vi "Contour Page.vi"() -> ()   [LabVIEW 2020, in "3D Contour.lvclass"]
uses:
  <vilib>/Math Plots/3D Math Plots/3D Contour/3D Contour/3D Contour.lvclass
  <vilib>/Math Plots/3D Math Plots/3D Contour/3D Contour/Typedef/3D Contour Property Array.ctl
  <vilib>/Math Plots/3D Math Plots/3D Contour/3D Contour/Typedef/3D Contour Property.ctl
  <vilib>/Math Plots/3D Math Plots/3D Plot/3D Plot/Typedef/Line Type.ctl
  <vilib>/Math Plots/3D Math Plots/3D Plot/3D Plot/Typedef/Color Ramp Cluster.ctl
  <vilib>/Math Plots/3D Math Plots/3D Plot/3D Plot/Typedef/Dialog State.ctl
  <vilib>/Math Plots/3D Math Plots/3D Plot/3D Plot/Typedef/Temp Scene State.ctl
  <vilib>/Math Plots/3D Math Plots/3D Plot/3D Plot/Typedef/Temp Scene Property Action.ctl
  <vilib>/Math Plots/3D Math Plots/3D Plot/3D Plot/3D Plot.lvclass
panel:
  out "Contour Property Out":T1
  in  "Contour Property In":T1
  in  "Interval":sgl min=0 step=0.001
  in  "Line Style":u16(ring) caption="Line style"
  in  "Antialiasing":bool
  in  "Line Width":sgl=0.001 caption="Line width" min=0.001 step=1
  in  "Line Color":u32(colorbox) caption="Line color"
  in  "Contour Mode":u16(ring) caption="Contour mode" items=["Contour", "Contour with surface"]
  in  "Axis Basis":u16(ring) caption="Axis basis" items=["X-Axis", "Y-Axis", "Z-Axis"]
  in  "Levels":u16=1 min=1 step=1
  in  "Level List":i32(listbox) caption="Level list"
  in  "Level Mode":u16(ring) caption="Level mode" items=["Levels", "Interval", "Level List"]
  in  "Ramp Edit":bool caption="Ramp edit"
  in  "Color Map Style":u16(ring) caption="Color map style" items=["None ", "Shaded", "Color spectrum", "Grey scale", "Custom"]
  out "Color Ramp":dbl[][](graph)
  in  "YZ Plane Projection":bool caption="YZ plane projection"
  in  "XZ Plane Projection":bool caption="XZ plane projection"
  in  "XY Plane Projection":bool caption="XY  plane projection"
  in  "Coordinate System":u16(ring) caption="Coordinate system" items=["Cartesian", "Cylindrical", "Spherical"]
  in  "Plot Opacity":sgl(slide) caption="Plot opacity(%)" min=0 max=100 scale=0.0..100.0
  in  "New":bool
  in  "Delete":bool
  in  "Move Up":bool
  in  "Move Down":bool
  in  "Plot List":i32(listbox)
  in  "Level Conflict":string="Can't have two contours have the same level."
  in  "New Line":string="[Add new level here]"
  in  "Event Registration":refnum<event-registration>
  # "Contour"
  # "General"
  # "Projection"
  # "Color Ramp"
  # "Contour"
  # "Line"
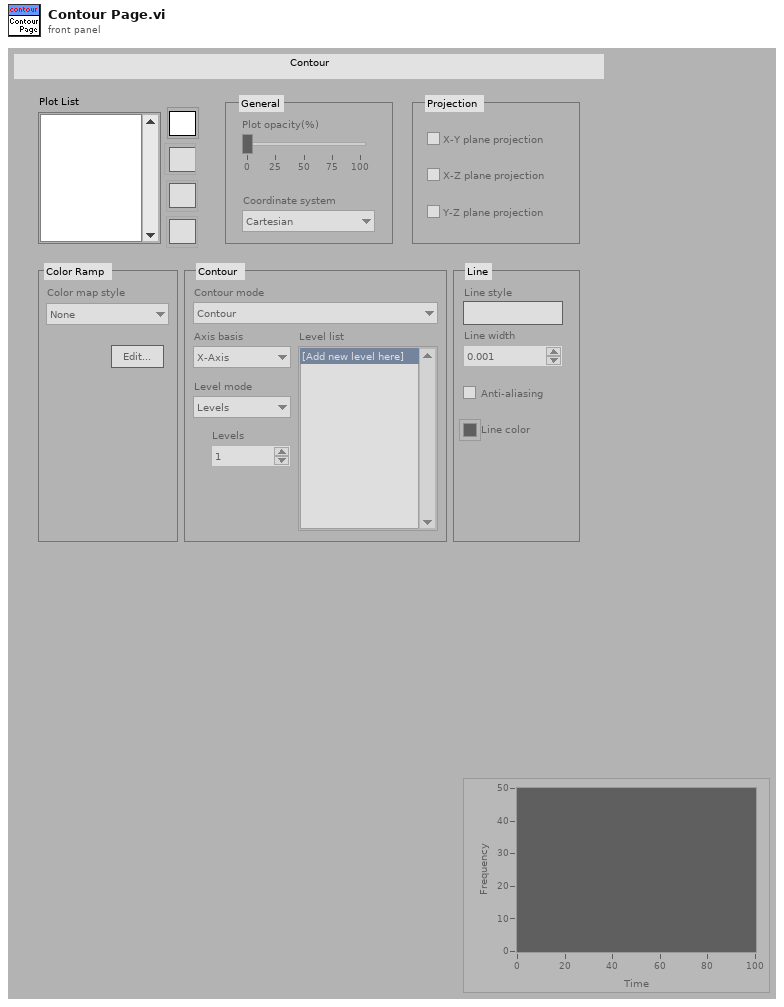
[diagram p1: front panel]
types:
  T1 = typedef "3D Contour.lvclass/3D Contour Property Array.ctl" = T2[]
  T2 = typedef "3D Contour.lvclass/3D Contour Property.ctl" = cluster{"General Property":cluster{"Plot Name":string, "Coordinate System":enum16{"Cartesian", "Cylindrical", "Spherical"}, "Opacity":sgl}, "Projection Property":cluster{"Draw XY":bool, "Draw YZ":bool, "Draw XZ":bool}, "Plot Property":cluster{"Line Style":T3, "Line Width":sgl, "Line Color":u32, "Antialiasing":bool, "Color Ramp Cluster":T4}, "Contour Property":cluster{"Contour Type":enum16{"Contour", "Contour with surface"}, "Axis Basis":enum16{"X-Axis", "Y-Axis", "Z-Axis"}, "Level List":sgl[], "Level Mode":enum16{"Levels", "Interval", "Level List"}, "Levels":u16, "Interval":sgl}}
  T3 = typedef "3D Plot.lvclass/Line Type.ctl" = enum16{"None", "Solid", "Dash", "Dot", "Dash Dot"}
  T4 = typedef "3D Plot.lvclass/Color Ramp Cluster.ctl" = cluster{"Color Ramp Style":enum16{"None", "Shaded", "Color spectrum", "Grey scale", "Custom"}, "Color Ramp Array":u32[], "Color Ramp Index":i32[], "Interpolate?":bool, "Logarithm?":bool}
  T5 = typedef "3D Plot.lvclass/Dialog State.ctl" = enum16{"Initialize", "Read Porperty", "Write Property", "Idle", "Exit"}
  T6 = typedef "3D Plot.lvclass/Temp Scene State.ctl" = enum16{"Create", "Update Scene", "Get Plot Representation", "Destory"}
  T7 = typedef "3D Plot.lvclass/Temp Scene Property Action.ctl" = enum16{"Graph Property", "Light Property", "Axis Property", "Value Pair Property", "Format Property", "Cursor Property", "Plot Specific Property"}
  T8 = typedef "3D Plot.lvclass/Multiplot Representation.ctl" = cluster{"Plot Represention Array":T9[], "Max Range":T10}
  T9 = typedef "3D Plot.lvclass/Plot Representation.ctl" = cluster{"Plot ID":i32, "Plot Range":T10, "Mesh Data":T11, "Dimension":cluster{"X Dimension":i32, "Y Dimension":i32}, "Ramp Range":T10}
  T10 = typedef "3D Plot.lvclass/Range Clusters.ctl" = cluster{"X Range":cluster{"Max X":sgl, "Min X":sgl}, "Y Range":cluster{"Max Y":sgl, "Min Y":sgl}, "Z Range":cluster{"Max Z":sgl, "Min Z":sgl}}
  T11 = typedef "3D Plot.lvclass/Mesh Data.ctl" = cluster{"Index Array":u32[], "Vertex Array":cluster{"X":sgl, "Y":sgl, "Z":sgl}[], "Normal Array":cluster{"X":sgl, "Y":sgl, "Z":sgl}[], "Color Index Array":i32[]}
  T12 = enum16{"None", "Shaded", "Color spectrum", "Grey scale", "Custom"}
  T13 = typedef "eventvkey.ctl" = enum16{"ASCII", "Enter", "Return", "Shift", "Ctrl", "Alt", "Cmd", "Opt", "Caps", "NumLock", "Clear", "Break", "Up", "Down", "Left", "Right", "Insert", "Delete", "Home", "End", "PageUp", "PageDown", "Escape", "Help", "Pause", "ScrollLock", "F1", "F2", "F3", "F4", "F5", "F6", "F7", "F8", "F9", "F10", "F11", "F12", "F13", "F14", "F15", "F16", "F17", "F18", "F19", "F20", "F21", "F22", "F23", "F24", "Play", "VolumeUp", "VolumeDown", "Mute", "Two Byte Char"}
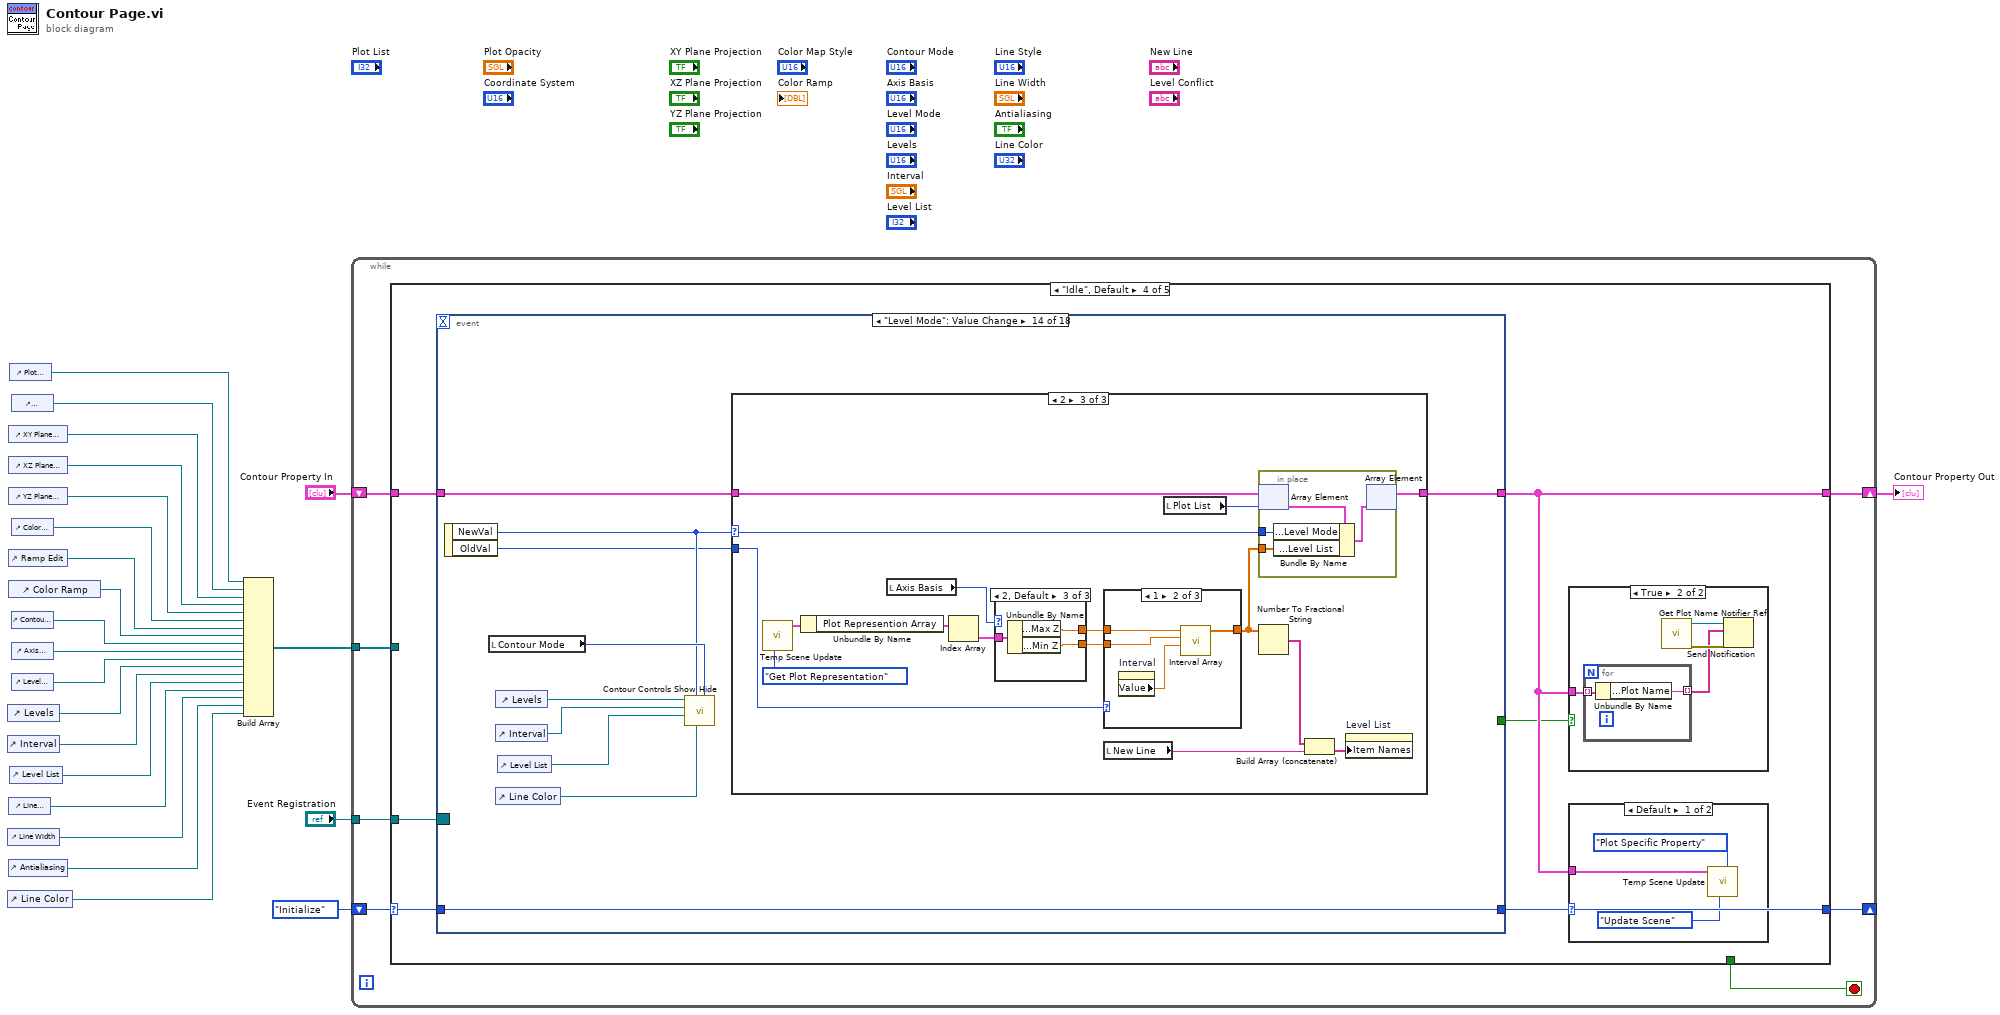
[diagram p0: block diagram]
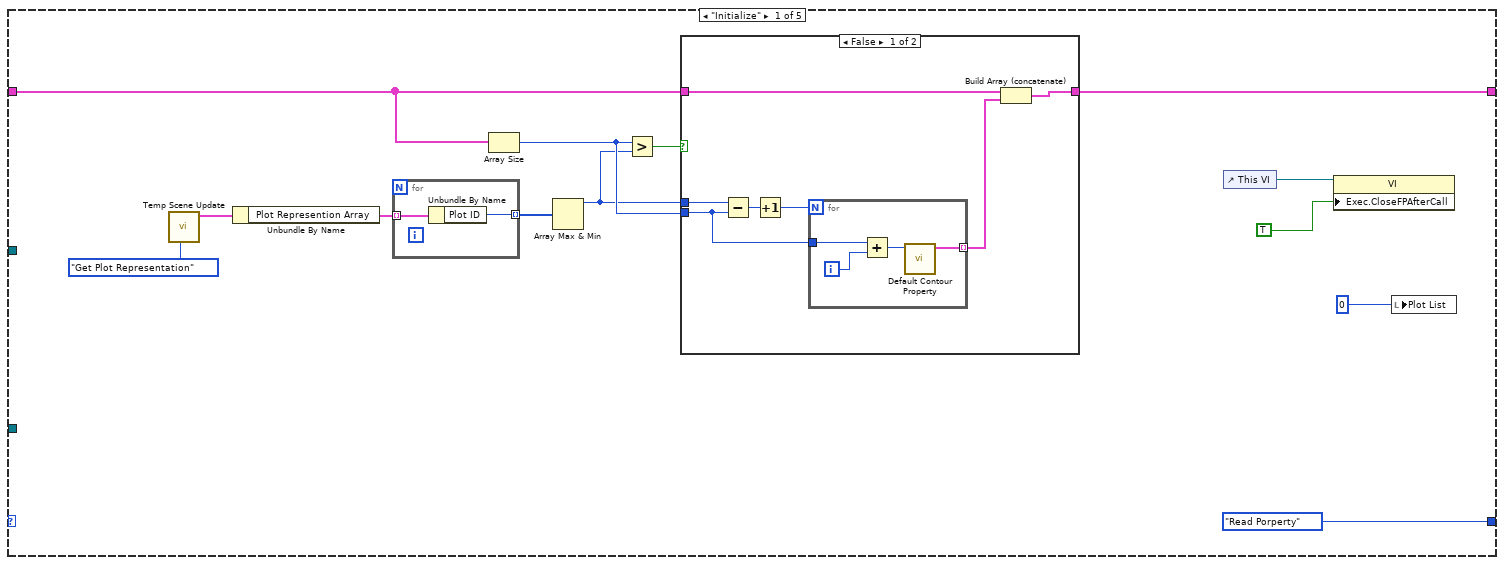
[diagram p2: hidden frame]
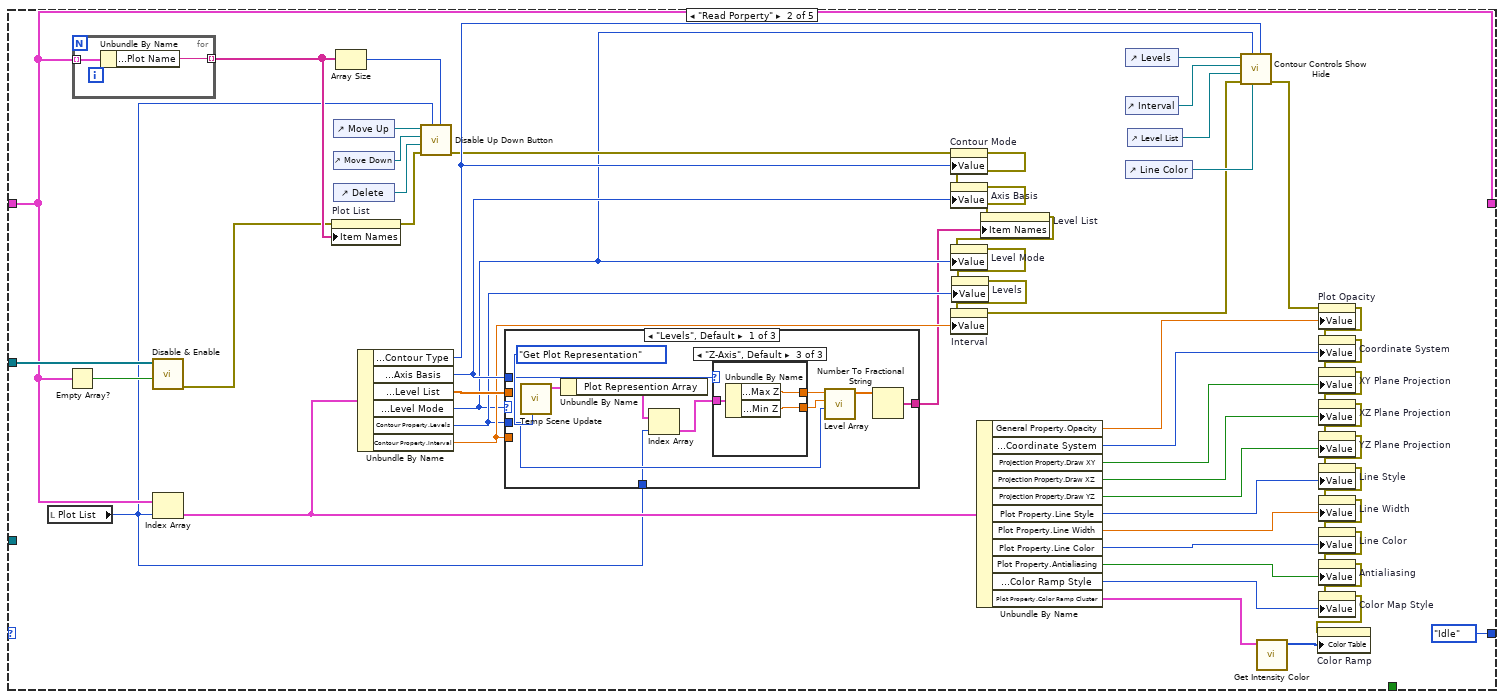
[diagram p4: hidden frame]
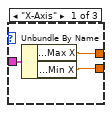
[diagram p5: hidden frame]
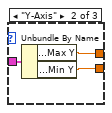
[diagram p6: hidden frame]
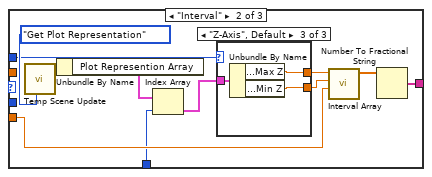
[diagram p7: hidden frame]
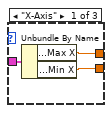
[diagram p8: hidden frame]
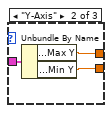
[diagram p9: hidden frame]
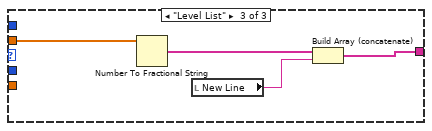
[diagram p10: hidden frame]
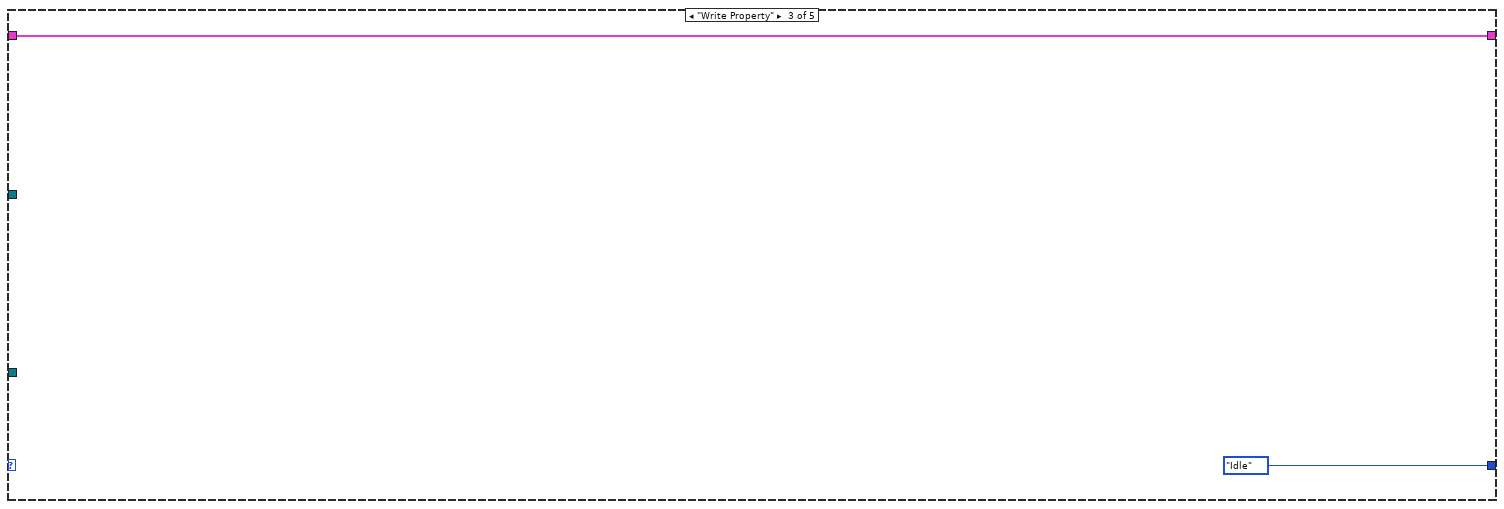
[diagram p11: hidden frame]
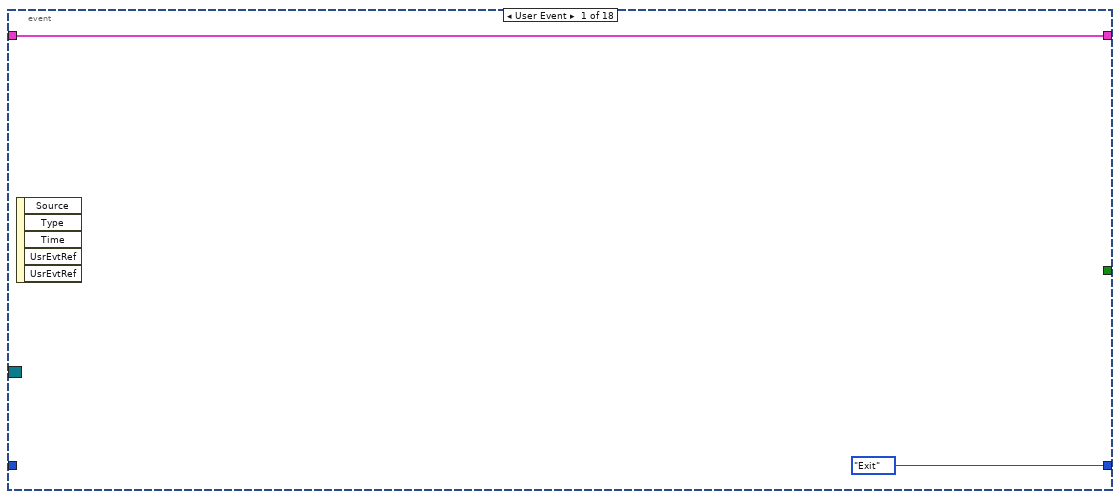
[diagram p14: hidden frame]
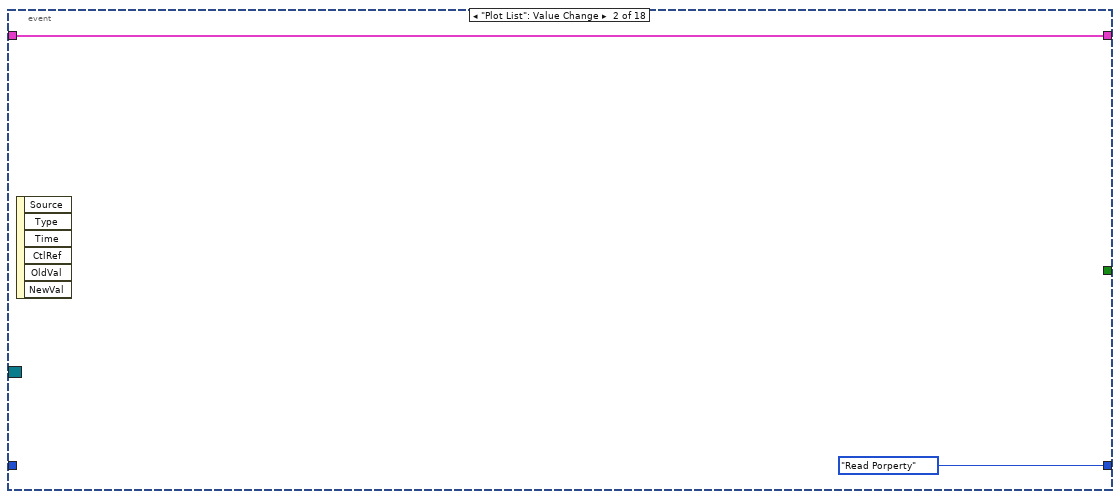
[diagram p15: hidden frame]
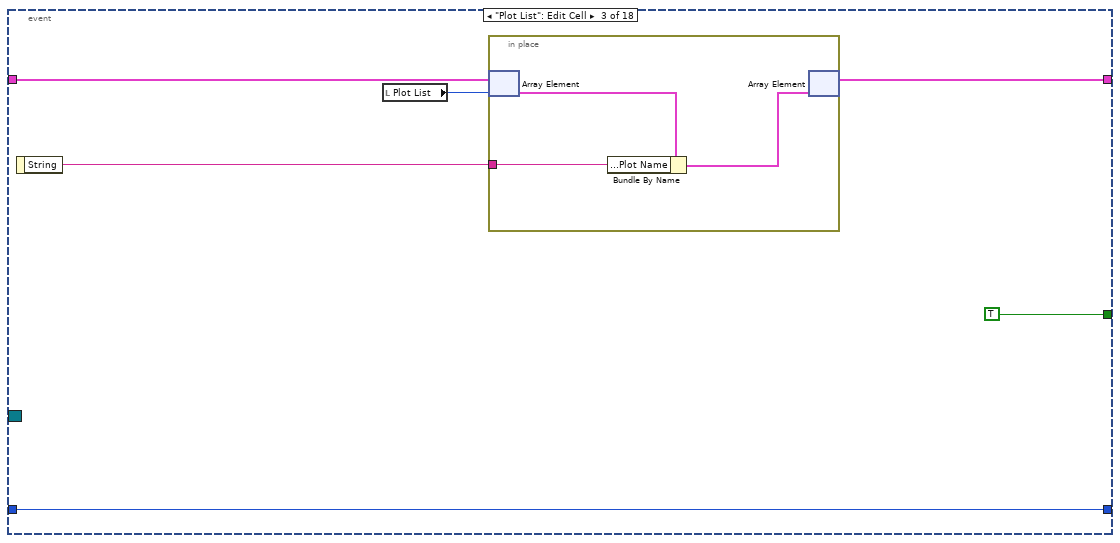
[diagram p16: hidden frame]
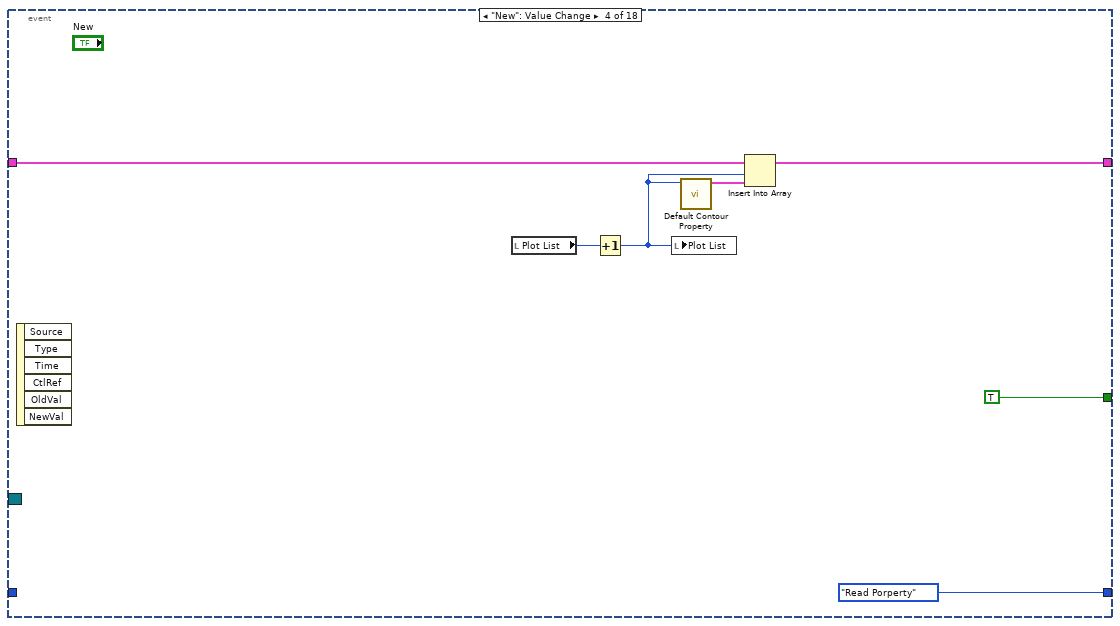
[diagram p17: hidden frame]
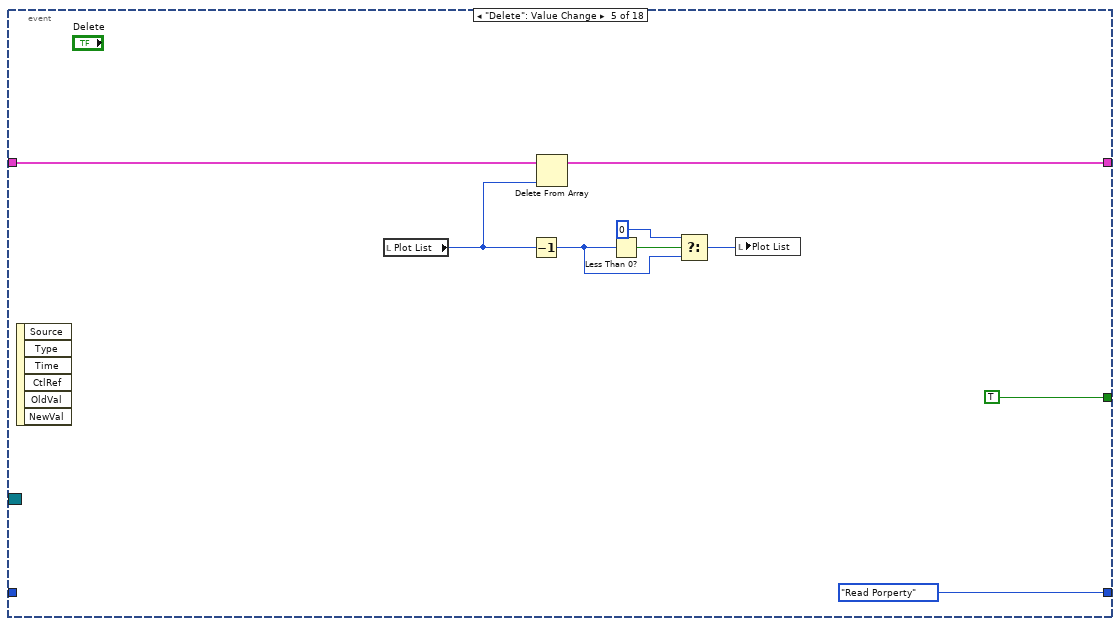
[diagram p18: hidden frame]
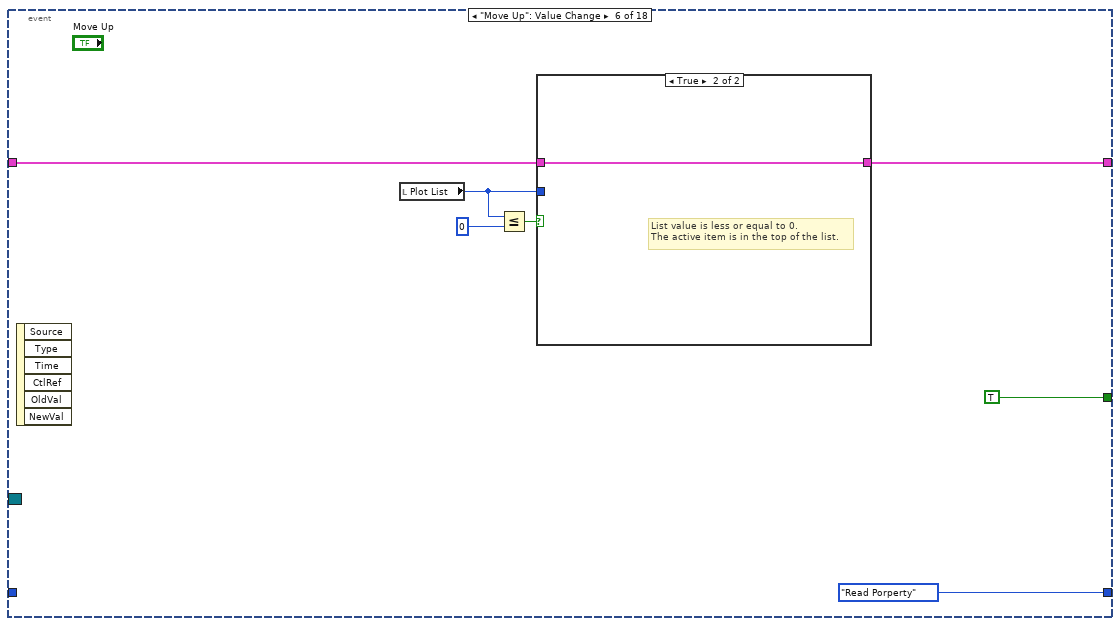
[diagram p19: hidden frame]
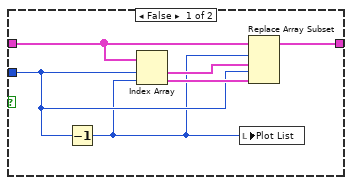
[diagram p20: hidden frame]
diagram:
  n1 = control-ref of="Levels"() -> (w8:refnum<vi>)
  n2 = control-ref of="Interval"() -> (w7:refnum<vi>)
  n3 = control-ref of="Line Width"() -> (w4:refnum<vi>)
  n4 = control-ref of="Line Color"() -> (w2:refnum<vi>)
  n5 = control-ref of="XY Plane Projection"() -> (w17:refnum<vi>)
  n6 = control-ref of="XZ Plane Projection"() -> (w16:refnum<vi>)
  n7 = control-ref of="YZ Plane Projection"() -> (w15:refnum<vi>)
  n8 = control-ref of="Ramp Edit"() -> (w13:refnum<vi>)
  n9 = control-ref of="Color Ramp"() -> (w12:refnum<vi>)
  n10 = control-ref of="Line Style"() -> (w5:refnum<vi>)
  n11 = control-ref of="Antialiasing"() -> (w3:refnum<vi>)
  n12 = control-ref of="Plot Opacity"() -> (w19:refnum<vi>)
  n13 = control-ref of="Level List"() -> (w6:refnum<vi>)
  n14 = control-ref of="Coordinate System"() -> (w18:refnum<vi>)
  n15 = control-ref of="Color Map Style"() -> (w14:refnum<vi>)
  n16 = control-ref of="Contour Mode"() -> (w11:refnum<vi>)
  n17 = control-ref of="Axis Basis"() -> (w10:refnum<vi>)
  n18 = control-ref of="Level Mode"() -> (w9:refnum<vi>)
  n19 = Build Array(w19, w18, w17, w16, w15, w14, w13, w12, w11, w10, w9, w8, w7, w6, w5, w4, w3, w2) -> (w1:refnum<vi>[])
  n20 = while {
    shift-right: [w29] -> w20
    shift-left: "Contour Property In" -> [w30]
    shift-right: [w25] -> _
    shift-left: Dialog_State."Initialize" -> [w28]
    tunnel: "Event Registration" -> [w26]
    tunnel: w1 -> [w24]
    stop <- w27 stop-if-true
    n21 = case shown="\"Idle\", Default" w28 {
      selector: w28 -> [_ _ _ w163 _]
      tunnel: w30 -> [w33 w96 w158 w165 w606]
      tunnel: [w32 w96 w158 w161 w606] -> w29
      tunnel: [Dialog_State."Read Porperty" Dialog_State."Idle" Dialog_State."Idle" w162 Dialog_State."Exit"] -> w25
      tunnel: [_ _ _ _ TRUE] -> w27
      tunnel: w26 -> [_ _ _ w164 _]
      tunnel: w24 -> [_ w97 _ _ _]
      frame "Initialize" {
        n22 = call <vilib>:"Temp Scene Update.vi"("State"=Temp_Scene_State."Get Plot Representation") -> ("Multiplot Representation"=w38:T8)  [unwired: 5 in, 5 out]
        n23 = Unbundle By Name(w38) -> ("Plot Represention Array"=w31:T9[])
        n24 = for {
          tunnel: w31 -> [w57] mode=indexing
          tunnel: [w56] -> w37 mode=indexing
          n25 = Unbundle By Name(w57) -> ("Plot ID"=w56:i32)
        }
        n26 = Array Size(array=w33) -> (size(s)=w35:i32)
        n27 = Array Max & Min(array=w37) -> (max value=w34:i32)  [unwired: 3 out]
        n28 = Greater?(x=w35, y=w34) -> (0:w36:bool)
        n29 = case shown="False" w36 {
          tunnel: [w48 w55] -> w32
          tunnel: w33 -> [w50 w55]
          tunnel: w35 -> [w44 _]
          tunnel: w34 -> [w45 _]
          frame False {
            n30 = Subtract(x=w45, y=w44) -> (x-y=w47:i32)
            n31 = Increment(x=w47) -> (x+1=w46:i32)
            n32 = for {
              N: w46 -> [_]
              tunnel: w44 -> [w53]
              tunnel: [w51] -> w49 mode=indexing
              i -> [w54]
              n33 = Add(x=w53, y=w54) -> (x+y=w52:i32)
              n34 = call <vilib>:"Default Contour Property.vi"("Plot ID"=w52) -> ("Default Property"=w51:T2)  [unwired: 10 out]
            }
            n35 = Build Array (concatenate)(w50, w49) -> (w48:T1)
          }
          frame True {
          }
        }
        n36 = control-ref of="This VI"() -> (w42:refnum<vi>)
        n37 = property class="VI"(reference=w42, "Exec.CloseFPAfterCall"=TRUE ("Execution:Close After Call")) -> ()  [unwired: 1 in, 2 out]
        n38 = local write "Plot List"(0 ("Plot List")) -> ()
      }
      frame "Read Porperty" {
        n39 = local read "Plot List"() -> (w59:i32)
        n40 = Empty Array?(array=w96) -> (empty?=w98:bool)
        n41 = for {
          tunnel: w96 -> [w157] mode=indexing
          tunnel: [w156] -> w104 mode=indexing
          n42 = Unbundle By Name(w157) -> ("General Property.Plot Name"=w156:string)
        }
        n43 = call <vilib>:"Disable & Enable.vi"("Disabled?"=w98, "Control Ref Array"=w97) -> ("error out"=w95:errorcluster)  [unwired: 1 in, 8 out]
        n44 = Index Array(array=w96, index=w59) -> (element=w110:T2)
        n45 = property on="Plot List" class="LstBox (strict)"(error in=w95, "Item Names"=w104) -> (error out=w103:errorcluster)  [unwired: 1 in, 1 out]
        n46 = control-ref of="Move Up"() -> (w106:refnum<vi>)
        n47 = control-ref of="Move Down"() -> (w107:refnum<vi>)
        n48 = control-ref of="Delete"() -> (w108:refnum<vi>)
        n49 = Array Size(array=w104) -> (size(s)=w105:i32)
        n50 = Unbundle By Name(w110) -> ("Contour Property.Contour Type"=w83:enum16{"Contour", "Contour with surface"}, "Contour Property.Axis Basis"=w64:enum16{"X-Axis", "Y-Axis", "Z-Axis"}, "Contour Property.Level List"=w65:sgl[], "Contour Property.Level Mode"=w61:enum16{"Levels", "Interval", "Level List"}, "Contour Property.Levels"=w62:u16, "Contour Property.Interval"=w63:sgl)
        n51 = call <vilib>:"Disable Up Down Button.vi"("Length"=w105, "Index"=w59, "error in (no error)"=w103, "Delete Ref"=w108, "Move Down Ref"=w107, "Move Up Ref"=w106) -> ("error out"=w69:errorcluster)  [unwired: 5 out]
        n52 = case shown="\"Levels\", Default" w61 {
          tunnel: [w114 w134 w152] -> w60
          tunnel: w65 -> [_ _ w155]
          tunnel: w64 -> [w117 w137 _]
          tunnel: w63 -> [_ w136 _]
          tunnel: w62 -> [w116 _ _]
          tunnel: w59 -> [w113 w133 _]
          frame "Levels", Default {
            n53 = call <vilib>:"Temp Scene Update.vi"("State"=Temp_Scene_State."Get Plot Representation") -> ("Multiplot Representation"=w118:T8)  [unwired: 5 in, 5 out]
            n54 = Unbundle By Name(w118) -> ("Plot Represention Array"=w112:T9[])
            n55 = Index Array(array=w112, index=w113) -> (element=w120:T9)
            n56 = case shown="\"Z-Axis\", Default" w117 {
              tunnel: w120 -> [w125 w128 w131]
              tunnel: [w124 w127 w130] -> w122
              tunnel: [w123 w126 w129] -> w121
              frame "X-Axis" {
                n57 = Unbundle By Name(w125) -> ("Plot Range.X Range.Max X"=w124:sgl, "Plot Range.X Range.Min X"=w123:sgl)
              }
              frame "Y-Axis" {
                n58 = Unbundle By Name(w128) -> ("Plot Range.Y Range.Max Y"=w127:sgl, "Plot Range.Y Range.Min Y"=w126:sgl)
              }
              frame "Z-Axis", Default {
                n59 = Unbundle By Name(w131) -> ("Plot Range.Z Range.Max Z"=w130:sgl, "Plot Range.Z Range.Min Z"=w129:sgl)
              }
            }
            n60 = call <vilib>:"Level Array.vi"("Level"=w116, "Min"=w121, "Max"=w122) -> ("Level Array"=w115:sgl[])  [unwired: 8 out]
            n61 = Number To Fractional String(number=w115) -> (F-format string=w114:string[])  [unwired: 3 out]
          }
          frame "Interval" {
            n62 = call <vilib>:"Temp Scene Update.vi"("State"=Temp_Scene_State."Get Plot Representation") -> ("Multiplot Representation"=w138:T8)  [unwired: 5 in, 5 out]
            n63 = Unbundle By Name(w138) -> ("Plot Represention Array"=w132:T9[])
            n64 = Index Array(array=w132, index=w133) -> (element=w140:T9)
            n65 = case shown="\"Z-Axis\", Default" w137 {
              tunnel: w140 -> [w145 w148 w151]
              tunnel: [w144 w147 w150] -> w142
              tunnel: [w143 w146 w149] -> w141
              frame "X-Axis" {
                n66 = Unbundle By Name(w145) -> ("Plot Range.X Range.Max X"=w144:sgl, "Plot Range.X Range.Min X"=w143:sgl)
              }
              frame "Y-Axis" {
                n67 = Unbundle By Name(w148) -> ("Plot Range.Y Range.Max Y"=w147:sgl, "Plot Range.Y Range.Min Y"=w146:sgl)
              }
              frame "Z-Axis", Default {
                n68 = Unbundle By Name(w151) -> ("Plot Range.Z Range.Max Z"=w150:sgl, "Plot Range.Z Range.Min Z"=w149:sgl)
              }
            }
            n69 = call <vilib>:"Interval Array.vi"("Interval"=w136, "Min"=w141, "Max"=w142) -> ("Level Array"=w135:sgl[])  [unwired: 8 out]
            n70 = Number To Fractional String(number=w135) -> (F-format string=w134:string[])  [unwired: 3 out]
          }
          frame "Level List" {
            n71 = Number To Fractional String(number=w155) -> (F-format string=w154:string[])  [unwired: 3 out]
            n72 = local read "New Line"() -> (w153:string)
            n73 = Build Array (concatenate)(w154, w153) -> (w152:string[])
          }
        }
        n74 = property on="Contour Mode" class="Ring (strict)"(error in=w69, "Value"=w83) -> (error out=w94:errorcluster)  [unwired: 1 in, 1 out]
        n75 = property on="Axis Basis" class="Ring (strict)"(error in=w94, "Value"=w64) -> (error out=w82:errorcluster)  [unwired: 1 in, 1 out]
        n76 = Unbundle By Name(w110) -> ("General Property.Opacity"=w81:sgl, "General Property.Coordinate System"=w80:enum16{"Cartesian", "Cylindrical", "Spherical"}, "Projection Property.Draw XY"=w79:bool, "Projection Property.Draw XZ"=w78:bool, "Projection Property.Draw YZ"=w77:bool, "Plot Property.Line Style"=w76:T3, "Plot Property.Line Width"=w75:sgl, "Plot Property.Line Color"=w74:u32, "Plot Property.Antialiasing"=w73:bool, "Plot Property.Color Ramp Cluster.Color Ramp Style"=w72:T12, "Plot Property.Color Ramp Cluster"=w58:T4)
        n77 = property on="Level List" class="LstBox (strict)"(error in=w82, "Item Names"=w60) -> (error out=w71:errorcluster)  [unwired: 1 in, 1 out]
        n78 = property on="Level Mode" class="Ring (strict)"(error in=w71, "Value"=w61) -> (error out=w93:errorcluster)  [unwired: 1 in, 1 out]
        n79 = property on="Levels" class="DigNum (strict)"(error in=w93, "Value"=w62) -> (error out=w92:errorcluster)  [unwired: 1 in, 1 out]
        n80 = property on="Interval" class="DigNum (strict)"(error in=w92, "Value"=w63) -> (error out=w70:errorcluster)  [unwired: 1 in, 1 out]
        n81 = control-ref of="Levels"() -> (w102:refnum<vi>)
        n82 = control-ref of="Interval"() -> (w101:refnum<vi>)
        n83 = control-ref of="Line Color"() -> (w99:refnum<vi>)
        n84 = control-ref of="Level List"() -> (w100:refnum<vi>)
        n85 = call <vilib>:"Contour Controls Show Hide.vi"("Contour Mode"=w83, "Line Color Ref"=w99, "Level Mode"=w61, "error in (no error)"=w70, "Level List Ref"=w100, "Interval Ref"=w101, "Levels Ref"=w102) -> ("error out"=w67:errorcluster)  [unwired: 4 out]
        n86 = call <vilib>:"Get Intensity Color.vi"("Color Ramp Cluster"=w58) -> ("Intensity Color"=w109:u32[])  [unwired: 4 in, 6 out]
        n87 = property on="Plot Opacity" class="Slide (strict)"(error in=w67, "Value"=w81) -> (error out=w91:errorcluster)  [unwired: 1 in, 1 out]
        n88 = property on="Coordinate System" class="Ring (strict)"(error in=w91, "Value"=w80) -> (error out=w90:errorcluster)  [unwired: 1 in, 1 out]
        n89 = property on="XY Plane Projection" class="Bool (strict)"(error in=w90, "Value"=w79) -> (error out=w89:errorcluster)  [unwired: 1 in, 1 out]
        n90 = property on="XZ Plane Projection" class="Bool (strict)"(error in=w89, "Value"=w78) -> (error out=w88:errorcluster)  [unwired: 1 in, 1 out]
        n91 = property on="YZ Plane Projection" class="Bool (strict)"(error in=w88, "Value"=w77) -> (error out=w87:errorcluster)  [unwired: 1 in, 1 out]
        n92 = property on="Line Style" class="Ring (strict)"(error in=w87, "Value"=w76) -> (error out=w86:errorcluster)  [unwired: 1 in, 1 out]
        n93 = property on="Line Width" class="DigNum (strict)"(error in=w86, "Value"=w75) -> (error out=w85:errorcluster)  [unwired: 1 in, 1 out]
        n94 = property on="Line Color" class="ColBox"(error in=w85, "Value"=w74) -> (error out=w84:errorcluster)  [unwired: 1 in, 1 out]
        n95 = property on="Antialiasing" class="Bool (strict)"(error in=w84, "Value"=w73) -> (error out=w68:errorcluster)  [unwired: 1 in, 1 out]
        n96 = property on="Color Map Style" class="Ring (strict)"(error in=w68, "Value"=w72) -> (error out=w66:errorcluster)  [unwired: 1 in, 1 out]
        n97 = property on="Color Ramp" class="IntGraph (strict)"(error in=w66, "Color Table"=w109) -> ()  [unwired: 1 in, 2 out]
      }
      frame "Write Property" {
      }
      frame "Idle", Default {
        n98 = event shown="[13] \"Level Mode\": Value Change" {
          selector: w164 -> [_ _ _ _ _ _ _ _ _ _ _ _ _ _ _ _ _ _]
          dyn-events: _ -> [_ _ _ _ _ _ _ _ _ _ _ _ _ _ _ _ _ _]
          timeout: _ -> [_ _ _ _ _ _ _ _ _ _ _ _ _ _ _ _ _ _]
          tunnel: w165 -> [w176 w178 w182 w192 w201 w206 w220 w234 w247 w266 w287 w303 w318 w353 w452 w477 w504 w563]
          tunnel: [w176 w178 w181 w191 w202 w205 w219 w233 w244 w265 w286 w302 w317 w352 w451 w478 w503 w562] -> w161
          tunnel: [Dialog_State."Exit" Dialog_State."Read Porperty" w180 Dialog_State."Read Porperty" Dialog_State."Read Porperty" Dialog_State."Read Porperty" Dialog_State."Read Porperty" w236 w248 w268 w289 w304 w319 w354 w457 w483 w505 w564] -> w162
          tunnel: w163 -> [_ _ w180 _ _ _ _ w236 w248 w268 w289 w304 w319 w354 w457 w483 w505 w564]
          tunnel: [_ _ TRUE TRUE TRUE TRUE TRUE _ _ _ _ _ _ _ _ _ _ _] -> w160
          event User Event {
            n99 = event-data() -> ()  [unwired: 6 out]
          }
          event "Plot List": Value Change {
            n100 = event-data() -> ()  [unwired: 7 out]
          }
          event "Plot List": Edit Cell {
            n101 = event-data() -> ("String"=w183:string)  [unwired: 1 out]
            n102 = local read "Plot List"() -> (w184:i32)
            n103 = in-place {
              in-place-border: w183 -> [w185]
              n104 = in-place-array #1(w182, w184) -> (w187:T2)
              n105 = Bundle By Name(cluster=w187, "General Property.Plot Name"=w185) -> (w186:T2)
              n106 = in-place-array #1(w186) -> (w181:T1)  [unwired: 1 out]
            }
          }
          event "New": Value Change {
            n107 = event-data() -> ()  [unwired: 7 out]
            n108 = local read "Plot List"() -> (w193:i32)
            n109 = Increment(x=w193) -> (x+1=w189:i32)
            n110 = local write "Plot List"(w189) -> ()
            n111 = call <vilib>:"Default Contour Property.vi"("Plot ID"=w189) -> ("Default Property"=w188:T2)  [unwired: 10 out]
            n112 = Insert Into Array(array=w192, index=w189, new element=w188) -> (w191:T1)
          }
          event "Delete": Value Change {
            n113 = event-data() -> ()  [unwired: 7 out]
            n114 = local read "Plot List"() -> (w197:i32)
            n115 = Decrement(x=w197) -> (x-1=w198:i32)
            n116 = Delete From Array(array=w201, index=w197) -> (array with subset deleted=w202:T1)  [unwired: 1 in, 1 out]
            n117 = Less Than 0?(x=w198) -> (x < 0?=w200:bool)
            n118 = Select(t=0, s=w200, f=w198) -> (s? t:f=w196:i32)
            n119 = local write "Plot List"(w196) -> ()
          }
          event "Move Up": Value Change {
            n120 = event-data() -> ()  [unwired: 7 out]
            n121 = local read "Plot List"() -> (w207:i32)
            n122 = Less Or Equal?(x=w207, y=0) -> (x <= y?=w208:bool)
            n123 = case shown="True" w208 {
              tunnel: w206 -> [w214 w217]
              tunnel: [w213 w217] -> w205
              tunnel: w207 -> [w212 _]
              frame False {
                n124 = Decrement(x=w212) -> (x-1=w211:i32)
                n125 = Index Array(array=w214, index #1=w212, index #2=w211) -> (element #1=w216:T2, element #2=w215:T2)
                n126 = local write "Plot List"(w211) -> ()
                n127 = Replace Array Subset(array=w214, new element #1=w216, index #1=w211, new element #2=w215, index #2=w212) -> (w213:T1)
              }
              frame True {
                # "List value is less or equal to 0.\nThe active item is in the top of the list."
              }
            }
          }
          event "Move Down": Value Change {
            n128 = event-data() -> ()  [unwired: 7 out]
            n129 = local read "Plot List"() -> (w221:i32)
            n130 = Increment(x=w221) -> (x+1=w223:i32)
            n131 = Array Size(array=w220) -> (size(s)=w224:i32)
            n132 = Greater?(x=w224, y=w223) -> (0:w222:bool)
            n133 = case shown="True" w222 {
              tunnel: w220 -> [w226 w230]
              tunnel: [w226 w229] -> w219
              tunnel: w221 -> [_ w228]
              frame False {
                # "List value +1 is not less array length.\nThe active item is in the buttom of the list."
              }
              frame True {
                n134 = Increment(x=w228) -> (x+1=w227:i32)
                n135 = Index Array(array=w230, index #1=w228, index #2=w227) -> (element #1=w232:T2, element #2=w231:T2)
                n136 = local write "Plot List"(w227) -> ()
                n137 = Replace Array Subset(array=w230, new element #1=w232, index #1=w227, new element #2=w231, index #2=w228) -> (w229:T1)
              }
            }
          }
          event "Plot Opacity", "Coordinate System", "XY Plane Projection", "XZ Plane Projection", "YZ Plane Projection": Value Change {
            n138 = event-data() -> ()  [unwired: 7 out]
            n139 = local read "Plot List"() -> (w235:i32)
            n140 = in-place {
              n141 = in-place-array #2(w234, w235) -> (w239:T2)
              n142 = local read "Coordinate System"() -> (w237:u16)
              n143 = local read "XY Plane Projection"() -> (w242:bool)
              n144 = local read "YZ Plane Projection"() -> (w240:bool)
              n145 = local read "XZ Plane Projection"() -> (w241:bool)
              n146 = local read "Plot Opacity"() -> (w243:sgl)
              n147 = Bundle By Name(cluster=w239, "General Property.Opacity"=w243, "General Property.Coordinate System"=w237, "Projection Property.Draw XY"=w242, "Projection Property.Draw YZ"=w240, "Projection Property.Draw XZ"=w241) -> (w238:T2)
              n148 = in-place-array #2(w238) -> (w233:T1)  [unwired: 1 out]
            }
          }
          event "Color Map Style": Value Change {
            n149 = event-data() -> ("NewVal"=w245:u16)  [unwired: 1 out]
            n150 = local read "Plot List"() -> (w246:i32)
            n151 = in-place {
              in-place-border: w245 -> [w250]
              n152 = in-place-array #3(w247, w246) -> (w251:T2)
              n153 = in-place {
                in-place-border: w250 -> [w255]
                n154 = in-place-cluster #4(w251) -> ("Plot Property.Color Ramp Cluster"=w256:T4)
                n155 = Bundle By Name(cluster=w256, "Color Ramp Style"=w255) -> (w254:T4)
                n156 = call <vilib>:"Regular Color Style.vi"("Color Ramp Cluster in"=w254) -> ("Color Ramp Cluster out"=w252:T4)  [unwired: 10 in]
                n157 = call <vilib>:"Get Intensity Color.vi"("Color Ramp Cluster"=w252) -> ("Intensity Color"=w253:u32[])  [unwired: 4 in, 6 out]
                n158 = property on="Color Ramp" class="IntGraph (strict)"("Color Table"=w253) -> ()  [unwired: 2 in, 2 out]
                n159 = in-place-cluster #4("Plot Property.Color Ramp Cluster"=w252) -> (w249:T2)
              }
              n160 = in-place-array #3(w249) -> (w244:T1)  [unwired: 1 out]
            }
          }
          event "Ramp Edit": Value Change {
            n161 = event-data() -> ()  [unwired: 7 out]
            n162 = call <vilib>:"Temp Scene Update.vi"("State"=Temp_Scene_State."Get Plot Representation") -> ("Multiplot Representation"=w262:T8)  [unwired: 5 in, 5 out]
            n163 = local read "Plot List"() -> (w267:i32)
            n164 = Unbundle By Name(w262) -> ("Plot Represention Array"=w257:T9[])
            n165 = local read "Plot List"() -> (w264:i32)
            n166 = local read "Axis Basis"() -> (w261:u16)
            n167 = Index Array(array=w257, index=w264) -> (element=w260:T9)
            n168 = case shown="2, Default" w261 {
              tunnel: w260 -> [w271 w274 w277]
              tunnel: [w270 w273 w276] -> w259
              tunnel: [w269 w272 w275] -> w258
              frame 0 {
                n169 = Unbundle By Name(w271) -> ("Plot Range.X Range.Max X"=w270:sgl, "Plot Range.X Range.Min X"=w269:sgl)
              }
              frame 1 {
                n170 = Unbundle By Name(w274) -> ("Plot Range.Y Range.Max Y"=w273:sgl, "Plot Range.Y Range.Min Y"=w272:sgl)
              }
              frame 2, Default {
                n171 = Unbundle By Name(w277) -> ("Plot Range.Z Range.Max Z"=w276:sgl, "Plot Range.Z Range.Min Z"=w275:sgl)
              }
            }
            n172 = in-place {
              in-place-border: w259 -> [w281]
              in-place-border: w258 -> [w280]
              n173 = in-place-array #5(w266, w267) -> (w284:T2)
              n174 = Unbundle By Name(w284) -> ("Plot Property.Color Ramp Cluster"=w283:T4)
              n175 = call <vilib>:"Color Editor.vi"("Min"=w280, "Max"=w281, "Color Ramp Cluster in"=w283) -> ("Color Ramp Cluster out"=w279:T4)  [unwired: 3 in, 5 out]
              n176 = Bundle By Name(cluster=w284, "Plot Property.Color Ramp Cluster"=w279) -> (w285:T2)
              n177 = Unbundle By Name(w279) -> ("Color Ramp Style"=w278:T12)
              n178 = call <vilib>:"Get Intensity Color.vi"("Color Ramp Cluster"=w279) -> ("Intensity Color"=w282:u32[])  [unwired: 4 in, 6 out]
              n179 = property on="Color Ramp" class="IntGraph (strict)"("Color Table"=w282) -> ()  [unwired: 2 in, 2 out]
              n180 = local write "Color Map Style"(w278) -> ()
              n181 = in-place-array #5(w285) -> (w265:T1)  [unwired: 1 out]
            }
          }
          event "Line Style", "Line Width", "Line Color", "Antialiasing": Value Change {
            n182 = event-data() -> ()  [unwired: 2 out]
            n183 = local read "Plot List"() -> (w288:i32)
            n184 = in-place {
              n185 = in-place-array #6(w287, w288) -> (w292:T2)
              n186 = local read "Line Color"() -> (w290:u32)
              n187 = local read "Antialiasing"() -> (w293:bool)
              n188 = local read "Line Width"() -> (w294:sgl)
              n189 = local read "Line Style"() -> (w295:u16)
              n190 = Bundle By Name(cluster=w292, "Plot Property.Line Style"=w295, "Plot Property.Line Width"=w294, "Plot Property.Line Color"=w290, "Plot Property.Antialiasing"=w293) -> (w291:T2)
              n191 = in-place-array #6(w291) -> (w286:T1)  [unwired: 1 out]
            }
          }
          event "Contour Mode": Value Change {
            n192 = event-data() -> ("NewVal"=w296:u16)  [unwired: 1 out]
            n193 = local read "Level Mode"() -> (w301:u16)
            n194 = control-ref of="Levels"() -> (w300:refnum<vi>)
            n195 = control-ref of="Interval"() -> (w299:refnum<vi>)
            n196 = control-ref of="Line Color"() -> (w297:refnum<vi>)
            n197 = control-ref of="Level List"() -> (w298:refnum<vi>)
            n198 = local read "Plot List"() -> (w305:i32)
            n199 = call <vilib>:"Contour Controls Show Hide.vi"("Contour Mode"=w296, "Line Color Ref"=w297, "Level Mode"=w301, "Level List Ref"=w298, "Interval Ref"=w299, "Levels Ref"=w300) -> ()  [unwired: 1 in, 5 out]
            n200 = in-place {
              in-place-border: w296 -> [w306]
              n201 = in-place-array #7(w303, w305) -> (w308:T2)
              n202 = Bundle By Name(cluster=w308, "Contour Property.Contour Type"=w306) -> (w307:T2)
              n203 = in-place-array #7(w307) -> (w302:T1)  [unwired: 1 out]
            }
          }
          event "Axis Basis": Value Change {
            n204 = event-data() -> ("NewVal"=w314:u16)  [unwired: 1 out]
            n205 = call <vilib>:"Temp Scene Update.vi"("State"=Temp_Scene_State."Get Plot Representation") -> ("Multiplot Representation"=w315:T8)  [unwired: 5 in, 5 out]
            n206 = Unbundle By Name(w315) -> ("Plot Represention Array"=w309:T9[])
            n207 = Index Array(array=w309) -> (element=w316:T9)  [unwired: 1 in]
            n208 = local read "Level Mode"() -> (w312:u16)
            n209 = case shown="2, Default" w314 {
              tunnel: w316 -> [w335 w338 w341]
              tunnel: [w334 w337 w340] -> w311
              tunnel: [w333 w336 w339] -> w310
              frame 0 {
                n210 = Unbundle By Name(w335) -> ("Plot Range.X Range.Max X"=w334:sgl, "Plot Range.X Range.Min X"=w333:sgl)
              }
              frame 1 {
                n211 = Unbundle By Name(w338) -> ("Plot Range.Y Range.Max Y"=w337:sgl, "Plot Range.Y Range.Min Y"=w336:sgl)
              }
              frame 2, Default {
                n212 = Unbundle By Name(w341) -> ("Plot Range.Z Range.Max Z"=w340:sgl, "Plot Range.Z Range.Min Z"=w339:sgl)
              }
            }
            n213 = local read "Plot List"() -> (w320:i32)
            n214 = case shown="0, Default" w312 {
              tunnel: w311 -> [w326 w332 _]
              tunnel: w310 -> [w325 w331 _]
              frame 0, Default {
                n215 = property on="Levels" class="DigNum (strict)"() -> (error out=w321:errorcluster, "Value"=w324:u16)  [unwired: 2 in, 1 out]
                n216 = call <vilib>:"Level Array.vi"("Level"=w324, "Min"=w325, "Max"=w326) -> ("Level Array"=w323:sgl[])  [unwired: 8 out]
                n217 = Number To Fractional String(number=w323) -> (F-format string=w322:string[])  [unwired: 3 out]
                n218 = property on="Level List" class="LstBox (strict)"(error in=w321, "Item Names"=w322) -> ()  [unwired: 1 in, 2 out]
              }
              frame 1 {
                n219 = property on="Interval" class="DigNum (strict)"() -> (error out=w327:errorcluster, "Value"=w330:sgl)  [unwired: 2 in, 1 out]
                n220 = call <vilib>:"Interval Array.vi"("Interval"=w330, "Min"=w331, "Max"=w332) -> ("Level Array"=w329:sgl[])  [unwired: 8 out]
                n221 = Number To Fractional String(number=w329) -> (F-format string=w328:string[])  [unwired: 3 out]
                n222 = property on="Level List" class="LstBox (strict)"(error in=w327, "Item Names"=w328) -> ()  [unwired: 1 in, 2 out]
              }
              frame 2 {
              }
            }
            n223 = in-place {
              in-place-border: w314 -> [w342]
              n224 = in-place-array #8(w318, w320) -> (w344:T2)
              n225 = Bundle By Name(cluster=w344, "Contour Property.Axis Basis"=w342) -> (w343:T2)
              n226 = in-place-array #8(w343) -> (w317:T1)  [unwired: 1 out]
            }
          }
          event "Level Mode": Value Change {
            n227 = event-data() -> ("NewVal"=w346:u16, "OldVal"=w345:u16)  [unwired: 1 out]
            n228 = local read "Contour Mode"() -> (w351:u16)
            n229 = control-ref of="Levels"() -> (w350:refnum<vi>)
            n230 = control-ref of="Interval"() -> (w349:refnum<vi>)
            n231 = control-ref of="Line Color"() -> (w347:refnum<vi>)
            n232 = control-ref of="Level List"() -> (w348:refnum<vi>)
            n233 = call <vilib>:"Contour Controls Show Hide.vi"("Contour Mode"=w351, "Line Color Ref"=w347, "Level Mode"=w346, "Level List Ref"=w348, "Interval Ref"=w349, "Levels Ref"=w350) -> ()  [unwired: 1 in, 5 out]
            n234 = case shown="2" w346 {
              selector: w346 -> [w362 w389 w423]
              tunnel: w353 -> [w361 w388 w422]
              tunnel: [w360 w387 w421] -> w352
              tunnel: w345 -> [_ _ w411]
              frame 0, Default {
                n235 = call <vilib>:"Temp Scene Update.vi"("State"=Temp_Scene_State."Get Plot Representation") -> ("Multiplot Representation"=w357:T8)  [unwired: 5 in, 5 out]
                n236 = Unbundle By Name(w357) -> ("Plot Represention Array"=w355:T9[])
                n237 = local read "Plot List"() -> (w365:i32)
                n238 = local read "Axis Basis"() -> (w367:u16)
                n239 = Index Array(array=w355, index=w365) -> (element=w359:T9)
                n240 = case shown="1" w367 {
                  tunnel: w359 -> [w372 w375 w378]
                  tunnel: [w371 w374 w377] -> w369
                  tunnel: [w370 w373 w376] -> w368
                  frame 0 {
                    n241 = Unbundle By Name(w372) -> ("Plot Range.X Range.Max X"=w371:sgl, "Plot Range.X Range.Min X"=w370:sgl)
                  }
                  frame 1 {
                    n242 = Unbundle By Name(w375) -> ("Plot Range.Y Range.Max Y"=w374:sgl, "Plot Range.Y Range.Min Y"=w373:sgl)
                  }
                  frame 2, Default {
                    n243 = Unbundle By Name(w378) -> ("Plot Range.Z Range.Max Z"=w377:sgl, "Plot Range.Z Range.Min Z"=w376:sgl)
                  }
                }
                n244 = property on="Levels" class="DigNum (strict)"() -> (error out=w356:errorcluster, "Value"=w364:u16)  [unwired: 2 in, 1 out]
                n245 = in-place {
                  in-place-border: w362 -> [w381]
                  n246 = in-place-array #9(w361, w365) -> (w380:T2)
                  n247 = Bundle By Name(cluster=w380, "Contour Property.Level Mode"=w381) -> (w379:T2)
                  n248 = in-place-array #9(w379) -> (w360:T1)  [unwired: 1 out]
                }
                n249 = call <vilib>:"Level Array.vi"("Level"=w364, "Min"=w368, "Max"=w369) -> ("Level Array"=w366:sgl[])  [unwired: 8 out]
                n250 = Number To Fractional String(number=w366) -> (F-format string=w363:string[])  [unwired: 3 out]
                n251 = property on="Level List" class="LstBox (strict)"(error in=w356, "Item Names"=w363) -> ()  [unwired: 1 in, 2 out]
              }
              frame 1 {
                n252 = call <vilib>:"Temp Scene Update.vi"("State"=Temp_Scene_State."Get Plot Representation") -> ("Multiplot Representation"=w384:T8)  [unwired: 5 in, 5 out]
                n253 = local read "Plot List"() -> (w392:i32)
                n254 = Unbundle By Name(w384) -> ("Plot Represention Array"=w382:T9[])
                n255 = local read "Axis Basis"() -> (w394:u16)
                n256 = Index Array(array=w382, index=w392) -> (element=w386:T9)
                n257 = case shown="0" w394 {
                  tunnel: w386 -> [w399 w402 w405]
                  tunnel: [w398 w401 w404] -> w396
                  tunnel: [w397 w400 w403] -> w395
                  frame 0 {
                    n258 = Unbundle By Name(w399) -> ("Plot Range.X Range.Max X"=w398:sgl, "Plot Range.X Range.Min X"=w397:sgl)
                  }
                  frame 1 {
                    n259 = Unbundle By Name(w402) -> ("Plot Range.Y Range.Max Y"=w401:sgl, "Plot Range.Y Range.Min Y"=w400:sgl)
                  }
                  frame 2, Default {
                    n260 = Unbundle By Name(w405) -> ("Plot Range.Z Range.Max Z"=w404:sgl, "Plot Range.Z Range.Min Z"=w403:sgl)
                  }
                }
                n261 = property on="Interval" class="DigNum (strict)"() -> (error out=w383:errorcluster, "Value"=w391:sgl)  [unwired: 2 in, 1 out]
                n262 = in-place {
                  in-place-border: w389 -> [w408]
                  n263 = in-place-array #10(w388, w392) -> (w407:T2)
                  n264 = Bundle By Name(cluster=w407, "Contour Property.Level Mode"=w408) -> (w406:T2)
                  n265 = in-place-array #10(w406) -> (w387:T1)  [unwired: 1 out]
                }
                n266 = call <vilib>:"Interval Array.vi"("Interval"=w391, "Min"=w395, "Max"=w396) -> ("Level Array"=w393:sgl[])  [unwired: 8 out]
                n267 = Number To Fractional String(number=w393) -> (F-format string=w390:string[])  [unwired: 3 out]
                n268 = property on="Level List" class="LstBox (strict)"(error in=w383, "Item Names"=w390) -> ()  [unwired: 1 in, 2 out]
              }
              frame 2 {
                n269 = call <vilib>:"Temp Scene Update.vi"("State"=Temp_Scene_State."Get Plot Representation") -> ("Multiplot Representation"=w417:T8)  [unwired: 5 in, 5 out]
                n270 = Unbundle By Name(w417) -> ("Plot Represention Array"=w409:T9[])
                n271 = local read "Axis Basis"() -> (w412:u16)
                n272 = Index Array(array=w409) -> (element=w418:T9)  [unwired: 1 in]
                n273 = case shown="2, Default" w412 {
                  tunnel: w418 -> [w436 w439 w442]
                  tunnel: [w435 w438 w441] -> w415
                  tunnel: [w434 w437 w440] -> w414
                  frame 0 {
                    n274 = Unbundle By Name(w436) -> ("Plot Range.X Range.Max X"=w435:sgl, "Plot Range.X Range.Min X"=w434:sgl)
                  }
                  frame 1 {
                    n275 = Unbundle By Name(w439) -> ("Plot Range.Y Range.Max Y"=w438:sgl, "Plot Range.Y Range.Min Y"=w437:sgl)
                  }
                  frame 2, Default {
                    n276 = Unbundle By Name(w442) -> ("Plot Range.Z Range.Max Z"=w441:sgl, "Plot Range.Z Range.Min Z"=w440:sgl)
                  }
                }
                n277 = case shown="1" w411 {
                  tunnel: w415 -> [w428 w432 _]
                  tunnel: w414 -> [w427 w431 _]
                  tunnel: [w425 w429 sgl[] [] ("Level Array")] -> w410
                  frame 0, Default {
                    n278 = property on="Levels" class="DigNum (strict)"() -> ("Value"=w426:u16)  [unwired: 2 in, 2 out]
                    n279 = call <vilib>:"Level Array.vi"("Level"=w426, "Min"=w427, "Max"=w428) -> ("Level Array"=w425:sgl[])  [unwired: 8 out]
                  }
                  frame 1 {
                    n280 = property on="Interval" class="DigNum (strict)"() -> ("Value"=w430:sgl)  [unwired: 2 in, 2 out]
                    n281 = call <vilib>:"Interval Array.vi"("Interval"=w430, "Min"=w431, "Max"=w432) -> ("Level Array"=w429:sgl[])  [unwired: 8 out]
                  }
                  frame 2 {
                  }
                }
                n282 = local read "New Line"() -> (w419:string)
                n283 = local read "Plot List"() -> (w424:i32)
                n284 = in-place {
                  in-place-border: w423 -> [w446]
                  in-place-border: w410 -> [w443]
                  n285 = in-place-array #11(w422, w424) -> (w444:T2)
                  n286 = Bundle By Name(cluster=w444, "Contour Property.Level Mode"=w446, "Contour Property.Level List"=w443) -> (w445:T2)
                  n287 = in-place-array #11(w445) -> (w421:T1)  [unwired: 1 out]
                }
                n288 = Number To Fractional String(number=w410) -> (F-format string=w413:string[])  [unwired: 3 out]
                n289 = Build Array (concatenate)(w413, w419) -> (w420:string[])
                n290 = property on="Level List" class="LstBox (strict)"("Item Names"=w420) -> ()  [unwired: 2 in, 2 out]
              }
            }
          }
          event "Levels": Value Change {
            n291 = event-data() -> ("NewVal"=w455:u16)  [unwired: 1 out]
            n292 = call <vilib>:"Temp Scene Update.vi"("State"=Temp_Scene_State."Get Plot Representation") -> ("Multiplot Representation"=w448:T8)  [unwired: 5 in, 5 out]
            n293 = Unbundle By Name(w448) -> ("Plot Represention Array"=w447:T9[])
            n294 = local read "Plot List"() -> (w454:i32)
            n295 = local read "Axis Basis"() -> (w460:u16)
            n296 = Index Array(array=w447, index=w454) -> (element=w450:T9)
            n297 = case shown="2, Default" w460 {
              tunnel: w450 -> [w463 w466 w469]
              tunnel: [w462 w465 w468] -> w459
              tunnel: [w461 w464 w467] -> w458
              frame 0 {
                n298 = Unbundle By Name(w463) -> ("Plot Range.X Range.Max X"=w462:sgl, "Plot Range.X Range.Min X"=w461:sgl)
              }
              frame 1 {
                n299 = Unbundle By Name(w466) -> ("Plot Range.Y Range.Max Y"=w465:sgl, "Plot Range.Y Range.Min Y"=w464:sgl)
              }
              frame 2, Default {
                n300 = Unbundle By Name(w469) -> ("Plot Range.Z Range.Max Z"=w468:sgl, "Plot Range.Z Range.Min Z"=w467:sgl)
              }
            }
            n301 = call <vilib>:"Level Array.vi"("Level"=w455, "Min"=w458, "Max"=w459) -> ("Level Array"=w456:sgl[])  [unwired: 8 out]
            n302 = in-place {
              in-place-border: w455 -> [w471]
              n303 = in-place-array #12(w452, w454) -> (w472:T2)
              n304 = Bundle By Name(cluster=w472, "Contour Property.Levels"=w471) -> (w470:T2)
              n305 = in-place-array #12(w470) -> (w451:T1)  [unwired: 1 out]
            }
            n306 = Number To Fractional String(number=w456) -> (F-format string=w453:string[])  [unwired: 3 out]
            n307 = property on="Level List" class="LstBox (strict)"("Item Names"=w453) -> ()  [unwired: 2 in, 2 out]
          }
          event "Interval": Value Change {
            n308 = event-data() -> ("NewVal"=w481:sgl)  [unwired: 1 out]
            n309 = call <vilib>:"Temp Scene Update.vi"("State"=Temp_Scene_State."Get Plot Representation") -> ("Multiplot Representation"=w474:T8)  [unwired: 5 in, 5 out]
            n310 = Unbundle By Name(w474) -> ("Plot Represention Array"=w473:T9[])
            n311 = local read "Plot List"() -> (w480:i32)
            n312 = local read "Axis Basis"() -> (w486:u16)
            n313 = Index Array(array=w473, index=w480) -> (element=w476:T9)
            n314 = case shown="1" w486 {
              tunnel: w476 -> [w489 w492 w495]
              tunnel: [w488 w491 w494] -> w485
              tunnel: [w487 w490 w493] -> w484
              frame 0 {
                n315 = Unbundle By Name(w489) -> ("Plot Range.X Range.Max X"=w488:sgl, "Plot Range.X Range.Min X"=w487:sgl)
              }
              frame 1 {
                n316 = Unbundle By Name(w492) -> ("Plot Range.Y Range.Max Y"=w491:sgl, "Plot Range.Y Range.Min Y"=w490:sgl)
              }
              frame 2, Default {
                n317 = Unbundle By Name(w495) -> ("Plot Range.Z Range.Max Z"=w494:sgl, "Plot Range.Z Range.Min Z"=w493:sgl)
              }
            }
            n318 = call <vilib>:"Interval Array.vi"("Interval"=w481, "Min"=w484, "Max"=w485) -> ("Level Array"=w482:sgl[])  [unwired: 8 out]
            n319 = in-place {
              in-place-border: w481 -> [w498]
              n320 = in-place-array #13(w477, w480) -> (w497:T2)
              n321 = Bundle By Name(cluster=w497, "Contour Property.Interval"=w498) -> (w496:T2)
              n322 = in-place-array #13(w496) -> (w478:T1)  [unwired: 1 out]
            }
            n323 = Number To Fractional String(number=w482) -> (F-format string=w479:string[])  [unwired: 3 out]
            n324 = property on="Level List" class="LstBox (strict)"("Item Names"=w479) -> ()  [unwired: 2 in, 2 out]
          }
          event "Level List": Edit Cell? {
            n325 = event-data() -> ("Row"=w507:i32, "String"=w500:string)  [unwired: 1 out]
            n326 = local read "New Line"() -> (w501:string)
            n327 = Equal?(x=w500, y=w501) -> (x = y?=w499:bool)
            n328 = case shown="False" w499 {
              tunnel: w500 -> [w510 w559]
              tunnel: w507 -> [w515 _]
              tunnel: [w514 TRUE ("Discard?")] -> w506
              tunnel: w504 -> [w513 w560]
              tunnel: [w512 w560] -> w503
              tunnel: [w511 w559] -> w502
              frame False {
                n329 = call <vilib>:"Trim Whitespace.vi"("string"=w510) -> ("trimmed string"=w509:string)  [unwired: 1 in]
                n330 = Empty String/Path?(string/path=w509) -> (empty?=w508:bool)
                n331 = case shown="False" w508 {
                  tunnel: w509 -> [w522 w557]
                  tunnel: w515 -> [w521 _]
                  tunnel: [w520 TRUE ("Discard?")] -> w514
                  tunnel: w513 -> [w519 w555]
                  tunnel: [w518 w555] -> w512
                  tunnel: [w516 w557] -> w511
                  frame False {
                    n332 = property on="Level List" class="LstBox (strict)"() -> ("Item Names"=w517:string[])  [unwired: 2 in, 2 out]
                    n333 = Fract/Exp String To Number(string=w522) -> (number=w523:dbl)  [unwired: 4 out]
                    n334 = Number To Fractional String(number=w523) -> (F-format string=w516:string)  [unwired: 3 out]
                    n335 = Search 1D Array(1D array=w517, element=w516) -> (index of element=w524:i32)  [unwired: 1 out]
                    n336 = case shown="-1" w524 {
                      selector: w524 -> [w528 _]
                      tunnel: [TRUE ("Discard?") FALSE ("Discard?")] -> w520
                      tunnel: w517 -> [_ w543]
                      tunnel: w521 -> [w529 w532]
                      tunnel: w519 -> [w525 w536]
                      tunnel: [w525 w535] -> w518
                      tunnel: w516 -> [_ w531]
                      frame Default {
                        n337 = Equal?(x=w528, y=w529) -> (x = y?=w527:bool)
                        n338 = case shown="False" w527 {
                          frame False {
                            n339 = local read "Level Conflict"() -> (w530:string)
                            n340 = One Button Dialog(message=w530) -> ()  [unwired: 2 out]
                          }
                          frame True {
                          }
                        }
                      }
                      frame -1 {
                        n341 = Array Size(array=w543) -> (size(s)=w541:i32)
                        n342 = Increment(x=w532) -> (x+1=w540:i32)
                        n343 = Replace Array Subset(array=w543, new element=w531, index=w532) -> (w533:string[])
                        n344 = Equal?(x=w541, y=w540) -> (x = y?=w542:bool)
                        n345 = case shown="True" w542 {
                          tunnel: w533 -> [w549 w553]
                          tunnel: [w548 w553] -> w539
                          frame False {
                            # "Edit existing value"
                            n346 = Array Size(array=w549) -> (size(s)=w551:i32)
                            n347 = Decrement(x=w551) -> (x-1=w550:i32)
                            n348 = Delete From Array(array=w549, index=w550) -> (array with subset deleted=w548:string[])  [unwired: 1 in, 1 out]
                          }
                          frame True {
                            # "Add a new value"
                            n349 = local read "New Line"() -> (w554:string)
                            n350 = Build Array (concatenate)(w553, w554) -> (w552:string[])
                            n351 = property on="Level List" class="LstBox (strict)"("Item Names"=w552) -> ()  [unwired: 2 in, 2 out]
                          }
                        }
                        n352 = local read "Plot List"() -> (w538:i32)
                        n353 = Fract/Exp String To Number(string=w539, default (0 dbl)=sgl 0.0 ("default (0 DBL)")) -> (number=w537:sgl[])  [unwired: 3 out]
                        n354 = in-place {
                          in-place-border: w537 -> [w545]
                          n355 = in-place-array #14(w536, w538) -> (w547:T2)
                          n356 = Bundle By Name(cluster=w547, "Contour Property.Level List"=w545) -> (w546:T2)
                          n357 = in-place-array #14(w546) -> (w535:T1)  [unwired: 1 out]
                        }
                      }
                    }
                  }
                  frame True {
                  }
                }
              }
              frame True {
              }
            }
            n358 = event-data("Discard?"=w506, "String"=w502) -> ()  [unwired: 1 in, 1 out]
          }
          event "Level List": Key Down? {
            n359 = event-data() -> ("Char"=w567:i16, "VKey"=w566:T13)  [unwired: 1 out]
            n360 = local read "Level Mode"() -> (w561:u16)
            n361 = case shown="2" w561 {
              tunnel: w567 -> [_ w574]
              tunnel: w566 -> [_ w573]
              tunnel: [FALSE w572] -> w565
              tunnel: w563 -> [w569 w571]
              tunnel: [w569 w570] -> w562
              frame Default {
                # "Levels and Intervals do not need to edit the list cell."
              }
              frame 2 {
                n362 = case shown="\"Delete\"" w573 {
                  tunnel: w574 -> [w577 _ _]
                  tunnel: [w576 FALSE FALSE] -> w572
                  tunnel: w571 -> [w575 w582 w604]
                  tunnel: [w575 w581 w604] -> w570
                  frame "ASCII" {
                    n363 = case shown="Default" w577 {
                      tunnel: [TRUE FALSE] -> w576
                      frame Default {
                        # "Igore other ASCII characters"
                      }
                      frame 8, 45, 46, 48..57 {
                        # "Back Space\n-\n.\n0~9\n\nare allowed"
                      }
                    }
                  }
                  frame "Delete" {
                    n364 = property on="Level List" class="LstBox (strict)"() -> (error out=w583:errorcluster, "Item Names"=w585:string[], "Value"=w584:i32)  [unwired: 2 in, 1 out]
                    n365 = Increment(x=w584) -> (x+1=w588:i32)
                    n366 = Delete From Array(array=w585, index=w584) -> (array with subset deleted=w589:string[])  [unwired: 1 in, 1 out]
                    n367 = Array Size(array=w585) -> (size(s)=w587:i32)
                    n368 = Equal?(x=w587, y=w588) -> (x = y?=w586:bool)
                    n369 = case shown="False" w586 {
                      tunnel: w589 -> [_ w591]
                      tunnel: w583 -> [_ w600]
                      tunnel: w582 -> [w590 w594]
                      tunnel: [w590 w593] -> w581
                      frame True {
                        # "New Lvl text can not be deleted"
                      }
                      frame False {
                        n370 = property on="Level List" class="LstBox (strict)"(error in=w600, "Item Names"=w591) -> ()  [unwired: 1 in, 2 out]
                        n371 = Array Size(array=w591) -> (size(s)=w599:i32)
                        n372 = local read "Plot List"() -> (w597:i32)
                        n373 = Decrement(x=w599) -> (x-1=w598:i32)
                        n374 = Delete From Array(array=w591, index=w598) -> (array with subset deleted=w592:string[])  [unwired: 1 in, 1 out]
                        n375 = Fract/Exp String To Number(string=w592, default (0 dbl)=sgl 0.0 ("default (0 DBL)")) -> (number=w596:sgl[])  [unwired: 3 out]
                        n376 = in-place {
                          in-place-border: w596 -> [w601]
                          n377 = in-place-array #15(w594, w597) -> (w603:T2)
                          n378 = Bundle By Name(cluster=w603, "Contour Property.Level List"=w601) -> (w602:T2)
                          n379 = in-place-array #15(w602) -> (w593:T1)  [unwired: 1 out]
                        }
                      }
                    }
                  }
                  frame Default {
                  }
                }
              }
            }
            n380 = event-data("Discard?"=w565) -> ()  [unwired: 1 in, 1 out]
          }
        }
        n381 = case shown="True" w160 {
          tunnel: w161 -> [_ w166]
          frame False {
          }
          frame True {
            n382 = for {
              tunnel: w166 -> [w171] mode=indexing
              tunnel: [w170] -> w167 mode=indexing
              n383 = Unbundle By Name(w171) -> ("General Property.Plot Name"=w170:string)
            }
            n384 = call <vilib>:"Get Plot Name Notifier Ref.vi"() -> ("error out"=w169:errorcluster, "Plot Names Notifier Ref"=w168:refnum<notifier>)  [unwired: 1 in, 9 out]
            n385 = Send Notification(notification=w167, notifier=w168, error in (no error)=w169) -> ()  [unwired: 2 out]
          }
        }
        n386 = case shown="Default" w162 {
          tunnel: w161 -> [w174 _]
          frame Default {
            n387 = call <vilib>:"Temp Scene Update.vi"("Property Name"=Temp_Scene_Property_Action."Plot Specific Property", "State"=Temp_Scene_State."Update Scene", "Property In"=w174) -> ()  [unwired: 3 in, 6 out]
          }
          frame "Exit" {
          }
        }
      }
      frame "Exit" {
      }
    }
  }
  "Contour Property Out" <- w20
